vi "BuildNyquist.vi"(9 "subset":cluster{"Min":dbl, "Max":dbl}={"Min"=0.0, "Max"=100000.0}, 11 "Complex FRF":cluster{"t0":dbl, "dt":dbl, "Y":cdb[]}) -> (0 "Phase":cluster{"t0":dbl, "dt":dbl, "Y":dbl[]}(graph), 1 "plots out":refnum<class "Base Datatype.lvclass">[](array[class]), 2 "Nyquist Plot":cluster{dbl[], dbl[]}(graph), 3 "Energy":cluster{"x0":dbl, "df":dbl, dbl[]}[](graph))   [LabVIEW 2022 SP3]
uses:
  <vilib>/Native 3D Graph/xcontrol/3DPC_SurfacePlot.xctl
  <vilib>/Native 3D Graph/classes/Base Datatype.lvclass
panel:
  out "Array":T1(array[cluster]) {"r" format="%.6f"}
  out "3D Nyquist":refnum<class "Base Datatype.lvclass">[](xcontrol)
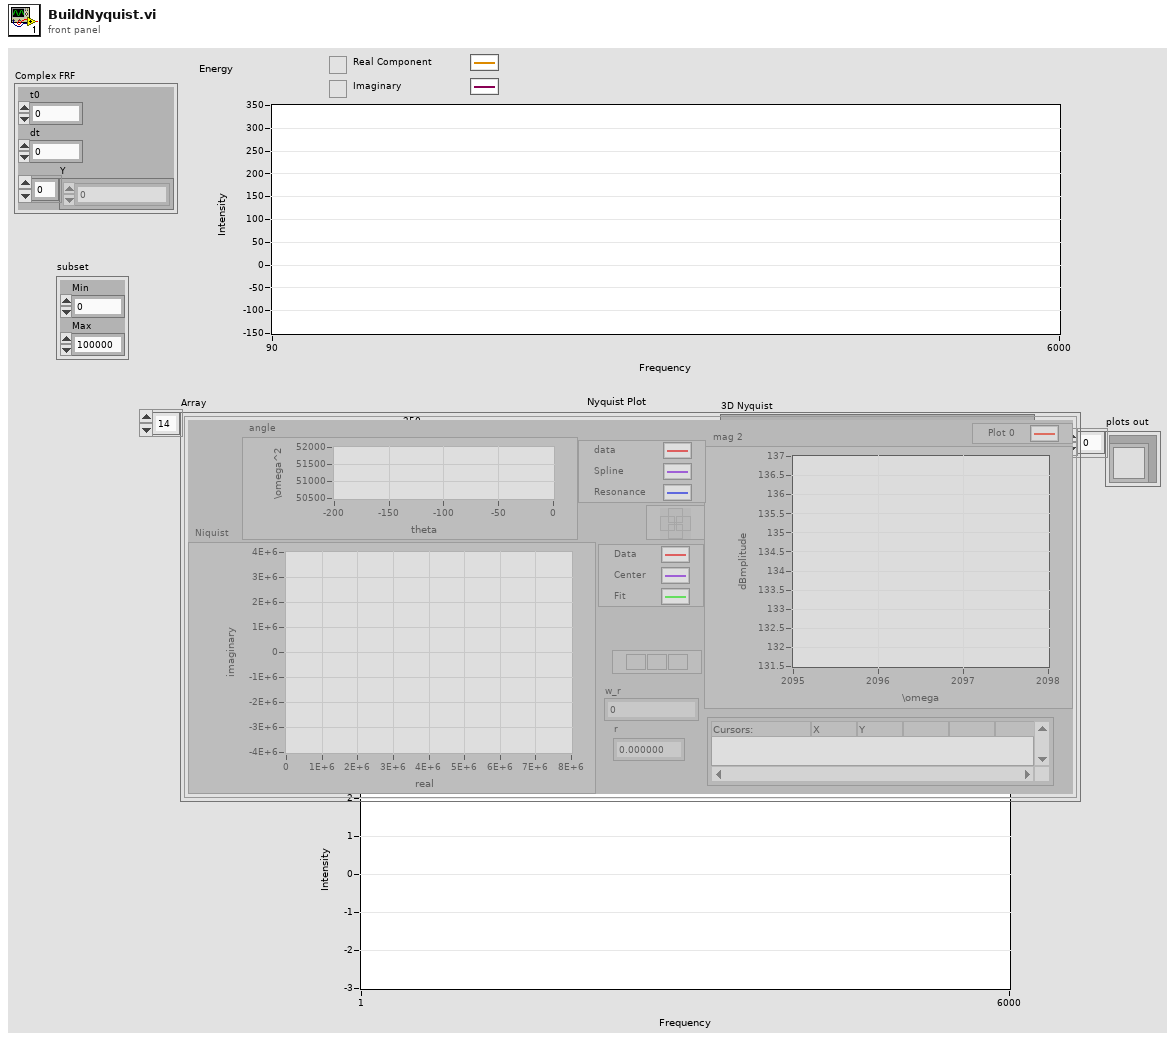
[diagram p1: front panel]
types:
  T1 = cluster{"angle":cluster{dbl[], "yi":dbl[]}[], "Niquist":cluster{dbl[], dbl[]}[], "mag 2":cluster{dbl[], dbl[]}, "w_r":dbl, "r":dbl}[]
  T2 = cluster{"angle":cluster{dbl[], "yi":dbl[]}[], "Niquist":cluster{dbl[], dbl[]}[], "mag 2":cluster{dbl[], dbl[]}, "w_r":dbl, "r":dbl}
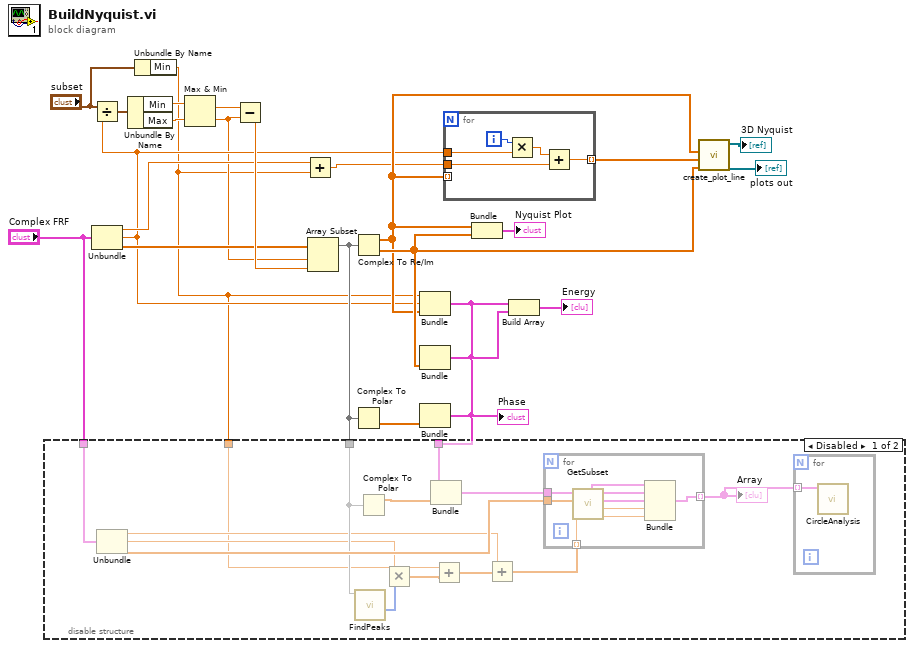
[diagram p0: block diagram]
diagram:
  n1 = Unbundle("Complex FRF") -> ("t0"=w11:dbl, "dt"=w6:dbl, "Y"=w12:cdb[])
  n2 = Divide(x="subset", y=w6) -> (x/y=w3:cluster{"Min":dbl, "Max":dbl})
  n3 = Unbundle By Name(w3) -> ("Min"=w4:dbl, "Max"=w15:dbl)
  n4 = Unbundle By Name("subset") -> ("Min"=w1:dbl)
  n5 = Max & Min(x=w4, y=w15) -> (max(x,y)=w14:dbl, min(x,y)=w5:dbl)
  n6 = Subtract(x=w14, y=w5) -> (x-y=w13:dbl)
  n7 = Add(x=w11, y=w1) -> (x+y=w7:dbl)
  n8 = Array Subset(array=w12, index=w5, length=w13) -> (w8:cdb[])
  n9 = Complex To Re/Im(x + iy=w8) -> (x=w17:dbl[], y=w18:dbl[])
  n10 = Complex To Polar(r * e^(i*theta)=w8) -> (theta=w23:dbl[])  [unwired: 1 out]
  n11 = Bundle("Min"=w1, "dt"=w6, w17) -> (w9:cluster{"Min":dbl, "dt":dbl, dbl[]})  [unwired: 1 in]
  n12 = disable-structure shown="Disabled" {
    disable-tunnel: "Complex FRF" -> [w36 _]
    disable-tunnel: w9 -> [w35 _]
    disable-tunnel: w8 -> [w33 _]
    disable-tunnel: w1 -> [w26 _]
    frame Disabled {
      n13 = Unbundle(w36) -> ("t0"=w31:dbl, "dt"=w32:dbl, "Y"=w38:cdb[])
      n14 = call "FindPeaks.vi"("subarray"=w33) -> ("indicies"=w29:i32[])  [unwired: 10 in]
      n15 = Complex To Polar(r * e^(i*theta)=w33) -> (r=w34:dbl[])  [unwired: 1 out]
      n16 = Multiply(x=w32, y=w29) -> (x*y=w28:dbl[])
      n17 = Bundle(cluster=w35, w34) -> (w37:cluster{"Min":dbl, "dt":dbl, dbl[]})  [unwired: 2 in]
      n18 = Add(x=w26, y=w28) -> (x+y=w27:dbl[])
      n19 = Add(x=w31, y=w27) -> (x+y=w30:dbl[])
      n20 = for {
        tunnel: w38 -> [w48]
        tunnel: w37 -> [w47]
        tunnel: w30 -> [w46] mode=indexing
        tunnel: [w45] -> w25 mode=indexing
        n21 = call "GetSubset.vi"("omega"=w46, "FFT"=w48, "mag"=w47) -> ("r"=w41:dbl, "w_r"=w42:dbl, "mag 2"=w43:cluster{dbl[], dbl[]}, "Niquist"=w44:cluster{dbl[], dbl[]}[], "angle"=w40:cluster{dbl[], "yi":dbl[]}[])  [unwired: 4 in]
        n22 = Bundle("angle"=w40, "Niquist"=w44, "mag 2"=w43, "w_r"=w42, "r"=w41) -> (w45:T2)  [unwired: 1 in]
      }
      "Array" <- w25
      n23 = for {
        tunnel: w25 -> [w39] mode=indexing
        n24 = call "CircleAnalysis.vi"("Cluster"=w39) -> ()  [unwired: 11 in]
      }
    }
    frame Enabled {
    }
  }
  n25 = Bundle(cluster=w9, w18) -> (w21:cluster{"Min":dbl, "dt":dbl, dbl[]})  [unwired: 2 in]
  n26 = Bundle(cluster=w9, w23) -> (→"Phase":cluster{"Min":dbl, "dt":dbl, dbl[]})  [unwired: 2 in]
  n27 = for {
    tunnel: w17 -> [_] mode=indexing
    tunnel: w6 -> [w52]
    tunnel: w7 -> [w50]
    tunnel: [w49] -> w19 mode=indexing
    i -> [w53]
    n28 = Multiply(x=w53, y=w52) -> (x*y=w51:dbl)
    n29 = Add(x=w51, y=w50) -> (x+y=w49:dbl)
  }
  n30 = Bundle(w17, w18) -> (→"Nyquist Plot":cluster{dbl[], dbl[]})  [unwired: 1 in]
  n31 = Build Array(w9, w21) -> (→"Energy":cluster{"Min":dbl, "dt":dbl, dbl[]}[])
  n32 = call <vilib>:"create_plot_line.vi"("z vector"=w18, "y vector"=w19, "x vector"=w17) -> ("plots out"=→"3D Nyquist" →"plots out":refnum<class "Base Datatype.lvclass">[])  [unwired: 2 in, 6 out]
